vi "CalculateSLERP.vi"(7 "t":dbl format="%#_13g", 9 "qb":T1, 11 "qa":T1) -> (3 "Quat (out)":T1)   [LabVIEW 2016]
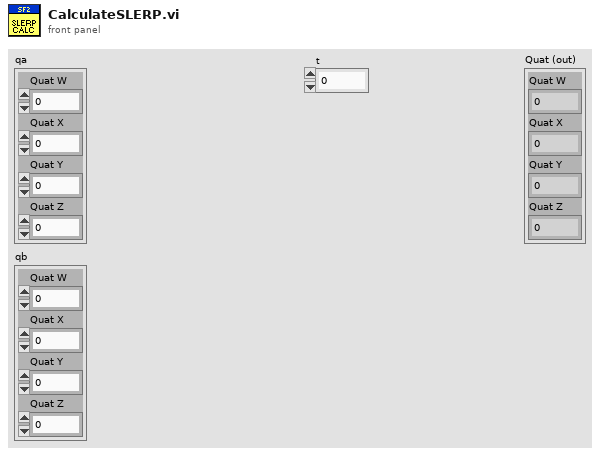
[diagram p1: front panel]
types:
  T1 = cluster{"Quat W":dbl, "Quat X":dbl, "Quat Y":dbl, "Quat Z":dbl}
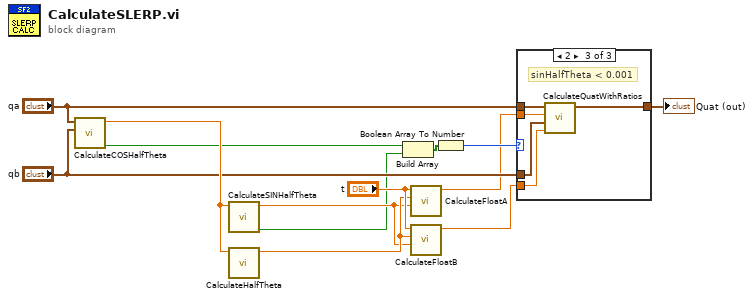
[diagram p0: block diagram]
diagram:
  n1 = call "CalculateCOSHalfTheta.vi"("qb"="qb", "qa"="qa") -> ("cosHalfTheta >= 1"=w6:bool, "cosHalfTheta"=w12:dbl)  [unwired: 8 in]
  n2 = call "CalculateSINHalfTheta.vi"("cosHalfTheta"=w12) -> ("sinHalfTheta < 0.001"=w5:bool, "sinHalfTheta"=w7:dbl)  [unwired: 9 in]
  n3 = call "CalculateHalfTheta.vi"("cosHalfTheta"=w12) -> ("HalfTheta"=w8:dbl)  [unwired: 10 in]
  n4 = Build Array(w6, w5) -> (w4:bool[])
  n5 = call "CalculateFloatA.vi"("sinHalfTheta"=w7, "HalfTheta"=w8, "t"="t") -> ("FloatRatioA"=w2:dbl)  [unwired: 8 in]
  n6 = call "CalculateFloatB.vi"("sinHalfTheta"=w7, "HalfTheta"=w8, "t"="t") -> ("FloatRatioB"=w1:dbl)  [unwired: 8 in]
  n7 = Boolean Array To Number(Boolean array=w4) -> (number=w3:u32)
  n8 = case shown="2" w3 {
    tunnel: "qa" -> [w14 w15 w20]
    tunnel: "qb" -> [_ _ w18]
    tunnel: [w14 w15 w19] -> w13
    tunnel: w2 -> [_ _ w17]
    tunnel: w1 -> [_ _ w16]
    frame 0, Default {
      # "Unknown"
    }
    frame 1 {
      # "cosHalfTheta >= 1"
    }
    frame 2 {
      # "sinHalfTheta < 0.001"
      n9 = call "CalculateQuatWithRatios.vi"("FloatRatioB"=w16, "qb (in)"=w18, "FloatRatioA"=w17, "qa (in)"=w20) -> ("Quat (out)"=w19:T1)  [unwired: 7 in]
    }
  }
  "Quat (out)" <- w13
